vi "SoundPlay.vi"(1 "Number of Samples/Iteration":i32=10000000, 2 "Volume":dbl(slide)=100.0 min=0.0 max=100.0 step=0.1 scale=0.0..100.0, 3 "Path to Sound file":path) -> (0 "error out":errorcluster)   [LabVIEW 2014]
doc: "This VI illustrates how to play a sound file continuously, reading the sound file in pieces, and playing each piece at a time."
uses:
  <vilib>/sound2/lvsound2.llb/Sampling Mode.ctl
  isPlaying.vi
  <vilib>/sound2/lvsound2.llb/Sound File Info (path).vi
  <vilib>/sound2/lvsound2.llb/Sound File Read Open.vi
  <vilib>/sound2/lvsound2.llb/Sound Output Set Volume (Single).vi
  <vilib>/sound2/lvsound2.llb/Sound File Read (DBL).vi
  <vilib>/sound2/lvsound2.llb/Sound Output Write (DBL).vi
panel:
  out "Numeric":dbl
  out "Current Data":waveform(dbl)[](graph)
  out "Current Iteration":i32
  in  "Stop":bool
  in  "Device ID":u32
  # "Overview: Demonstrates the use of the Sound VIs to play a sound file continuously, reading the sound file in pieces, and playing each piece one at a time.\nInstructions:\n1. Specify the Device ID and the Number of Samples/Iteration.\n2. Run the VI."
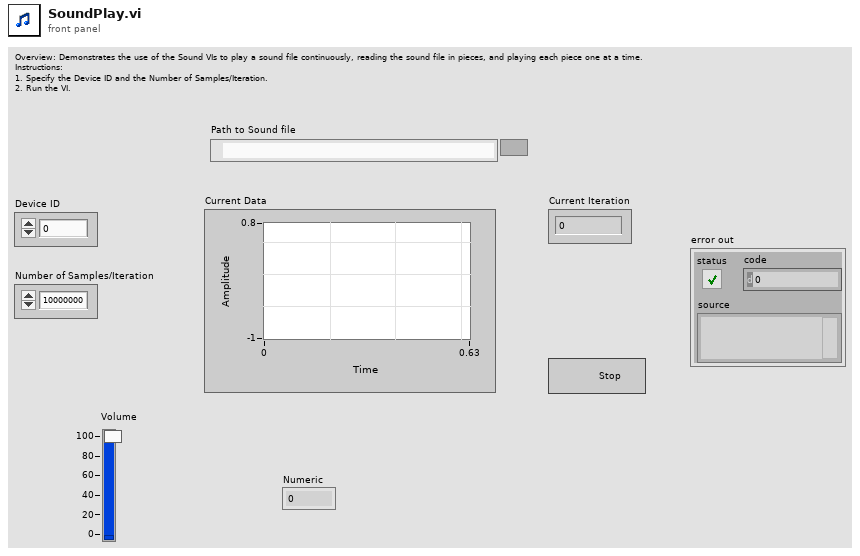
[diagram p1: front panel]
types:
  T1 = typedef "Sampling Mode.ctl" = i32
  T2 = typedef "Sound Data Format.ctl" = cluster{"sample rate (S/s)":dbl, "number of channels":i32, "bits per sample":i32}
  T3 = typedef "Sound File Refnum.ctl" = refnum<file>
  T4 = typedef "Sound Output Task ID.ctl" = u32
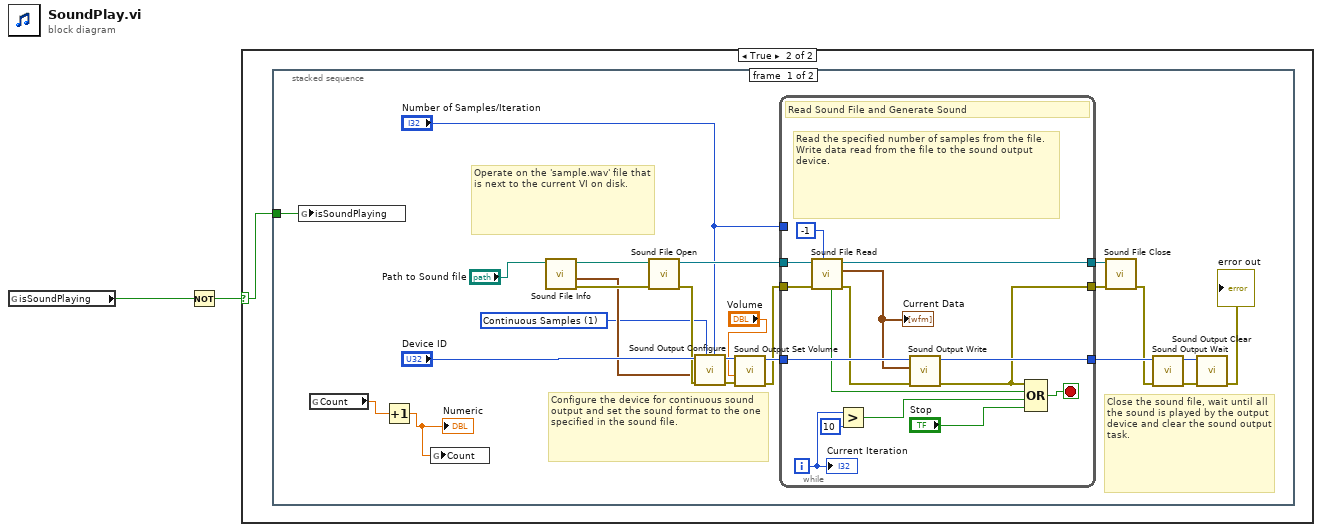
[diagram p0: block diagram]
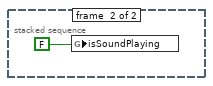
[diagram p3: hidden frame]
diagram:
  n1 = global read "isPlaying.vi" "isSoundPlaying"() -> (w2:bool)
  n2 = Not(x=w2) -> (.not. x?=w1:bool)
  n3 = case shown="True" w1 {
    selector: w1 -> [_ w3]
    frame False {
    }
    frame True {
      n4 = stacked-sequence {
        tunnel: w3 -> [w6 _]
        frame #0 {
          w14 = T1 1 items=["Finite Samples", "Continuous Samples"] ("sample mode")
          # "Operate on the 'sample.wav' file that is next to the current VI on disk."
          # "Close the sound file, wait until all the sound is played by the output device and clear the sound output task."
          # "Configure the device for continuous sound output and set the sound format to the one specified in the sound file."
          n5 = global write "isPlaying.vi" "isSoundPlaying"(w6) -> ()
          n6 = global read "isPlaying.vi" "Count"() -> (w5:dbl)
          n7 = Increment(x=w5) -> (x+1=w4:dbl)
          "Numeric" <- w4
          n8 = global write "isPlaying.vi" "Count"(w4) -> ()
          n9 = call-poly <vilib>:"Sound File Info.vi"("path"="Path to Sound file") -> ("error out"=w23:errorcluster, "sound format"=w16:T2, "path out"=w17:path)  [unwired: 7 in, 1 out]
          n10 = call-poly <vilib>:"Sound File Open.vi"("error in (no error)"=w23, "path"=w17) -> ("error out"=w22:errorcluster, "sound file refnum"=w24:T3)  [unwired: 8 in]
          n11 = call <vilib>:"Sound Output Configure.vi"("number of samples/ch"="Number of Samples/Iteration", "sample mode"=w14, "error in (no error)"=w22, "sound format"=w16, "device ID"="Device ID") -> ("error out"=w10:errorcluster, "task ID"=w11:T4)  [unwired: 5 in]
          n12 = call-poly <vilib>:"Sound Output Set Volume.vi"("error in (no error)"=w10, "volume"="Volume", "task ID"=w11) -> ("error out"=w8:errorcluster, "task ID out"=w9:T4)  [unwired: 7 in]
          n13 = while {
            tunnel: "Number of Samples/Iteration" -> [_]
            tunnel: w24 -> [w40]
            tunnel: [w39] -> w26
            tunnel: w8 -> [w41]
            tunnel: [w34] -> w25
            tunnel: w9 -> [w38]
            tunnel: [w42] -> w20
            i -> [w32]
            stop <- w35 stop-if-true
            # "Read the specified number of samples from the file. Write data read from the file to the sound output device."
            # "Read Sound File and Generate Sound"
            n14 = call-poly <vilib>:"Sound File Read.vi"("number of samples/ch (-1: all)"=-1, "error in (no error)"=w41, "sound file refnum"=w40) -> ("error out"=w37:errorcluster, "data"=w33:waveform(dbl)[], "sound file refnum out"=w39:T3, "end of file?"=w36:bool)  [unwired: 4 in, 1 out]
            "Current Data" <- w33
            n15 = Greater?(x=w32, y=10) -> (0:w29:bool)
            n16 = call-poly <vilib>:"Sound Output Write.vi"("error in (no error)"=w37, "data"=w33, "task ID"=w38) -> ("error out"=w34:errorcluster, "task ID out"=w42:T4)  [unwired: 7 in]
            n17 = Compound Arithmetic op=OR(w34, w36, w29, "Stop") -> (w35:bool)
            "Current Iteration" <- w32
          }
          n18 = call <vilib>:"Sound File Close.vi"("error in (no error)"=w25, "sound file refnum"=w26) -> ("error out"=w19:errorcluster)  [unwired: 9 in]
          n19 = call <vilib>:"Sound Output Wait.vi"("error in (no error)"=w19, "task ID"=w20) -> ("error out"=w18:errorcluster, "task ID out"=w21:T4)  [unwired: 8 in]
          n20 = call <vilib>:"Sound Output Clear.vi"("error in (no error)"=w18, "task ID"=w21) -> ("error out"=→"error out":errorcluster)  [unwired: 9 in]
        }
        frame #1 {
          n21 = global write "isPlaying.vi" "isSoundPlaying"(FALSE) -> ()
        }
      }
    }
  }
